vi "CH_LM VI Tree.vi"   [LabVIEW 2012, in "CH_LM.lvlib"]
doc: "This is the instrument driver for Coherent's <B>LabMax</B>. The VI Tree displays all the user-callable VIs of the instrument driver in an organized table."
uses:
  CH_LM.lvlib
  CH_LM Display Mode.ctl
  CH_LM Communication Mode.ctl
panel:
  # "(c) 2007 Coherent Inc.  ALL RIGHTS RESERVED."
  # "SEE DIAGRAM\nFOR VI TREE."
types:
  T1 = typedef "CH_LM.lvlib/CH_LM Communication Mode.ctl" = enum16{"None", "USB", "GPIB", "RS232"}
  T2 = typedef "CH_LM.lvlib/CH_LM Display Mode.ctl" = enum16{"Non-Statistics", "Statistics", "Position Stability", "Tune", "Trend"}
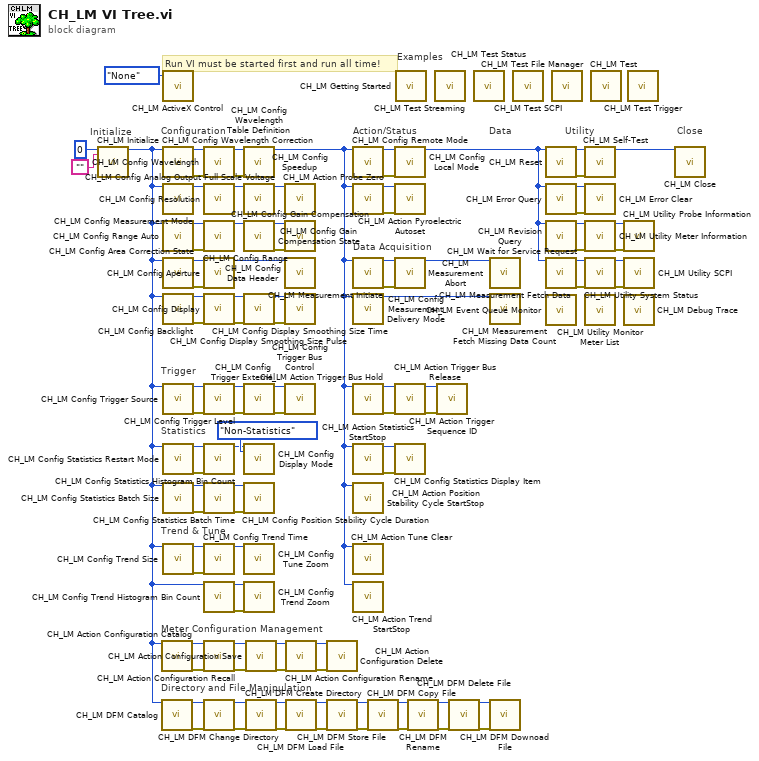
[diagram p0: block diagram]
diagram:
  # "Data Acquisition"
  # "Trigger"
  # "Statistics"
  # "Trend & Tune"
  # "Directory and File Manipulation"
  # "Meter Configuration Management"
  # "Run VI must be started first and run all time!"
  # "Examples"
  # "Configuration"
  # "Utility"
  # "Data"
  # "Action/Status"
  # "Close"
  # "Initialize"
  n1 = call "CH_LM Initialize.vi"("Address"=0, "Serial Number"="") -> ("Meter Index"=w5:i32)  [unwired: 3 in, 14 out]
  n2 = call "CH_LM Action Configuration Catalog.vi"("Meter Index"=w5) -> ("Meter Index"=w61:i32, "error out"=w60:errorcluster)  [unwired: 1 in, 16 out]
  n3 = call "CH_LM DFM Catalog.vi"("Meter Index"=w5) -> ("Meter Index"=w27:i32, "error out"=w24:errorcluster)  [unwired: 1 in, 16 out]
  n4 = call "CH_LM ActiveX Control.vi"("Communication Mode"=CH_LM_Communication_Mode."None") -> ()  [unwired: 3 in, 2 out]
  n5 = call "CH_LM Config Wavelength Correction.vi"("Meter Index"=w5) -> ("Meter Index"=w76:i32, "error out"=w9:errorcluster)  [unwired: 3 in, 14 out]
  n6 = call "CH_LM Config Measurement Mode.vi"("Meter Index"=w5) -> ("Meter Index"=w63:i32)  [unwired: 4 in, 14 out]
  n7 = call "CH_LM Config Range Auto.vi"("Meter Index"=w5) -> ("Meter Index"=w37:i32, "error out"=w11:errorcluster)  [unwired: 3 in, 14 out]
  n8 = call "CH_LM Config Area Correction State.vi"("Meter Index"=w5) -> ("Meter Index"=w73:i32, "error out"=w72:errorcluster)  [unwired: 3 in, 14 out]
  n9 = call "CH_LM Config Backlight.vi"("Meter Index"=w5) -> ("Meter Index"=w79:i32, "error out"=w78:errorcluster)  [unwired: 7 in, 10 out]
  n10 = call "CH_LM Config Trigger Source.vi"("Meter Index"=w5) -> ("Meter Index"=w45:i32, "error out"=w44:errorcluster)  [unwired: 3 in, 14 out]
  n11 = call "CH_LM Config Statistics Restart Mode.vi"("Meter Index"=w5) -> ("Meter Index"=w67:i32, "error out"=w66:errorcluster)  [unwired: 3 in, 14 out]
  n12 = call "CH_LM Config Statistics Batch Size.vi"("Meter Index"=w5) -> ("Meter Index"=w64:i32, "error out"=w65:errorcluster)  [unwired: 4 in, 13 out]
  n13 = call "CH_LM Config Trend Size.vi"("Meter Index"=w5) -> ("Meter Index"=w33:i32, "error out"=w7:errorcluster)  [unwired: 4 in, 13 out]
  n14 = call "CH_LM Config Wavelength.vi"("Meter Index"=w76, "error in (no error)"=w9) -> ("Meter Index"=w70:i32, "error out"=w10:errorcluster)  [unwired: 3 in, 13 out]
  n15 = call "CH_LM Config Resolution.vi"("Meter Index"=w63) -> ("Meter Index"=w31:i32)  [unwired: 4 in, 14 out]
  n16 = call "CH_LM Config Range.vi"("Meter Index"=w37, "error in (no error)"=w11) -> ("Meter Index"=w32:i32)  [unwired: 3 in, 14 out]
  n17 = call "CH_LM Config Aperture.vi"("Meter Index"=w73, "error in (no error)"=w72) -> ("Meter Index"=w2:i32)  [unwired: 2 in, 15 out]
  n18 = call "CH_LM Config Display.vi"("Meter Index"=w79, "error in (no error)"=w78) -> ("Meter Index"=w4:i32, "error out"=w3:errorcluster)  [unwired: 4 in, 12 out]
  n19 = call "CH_LM Config Trigger Level.vi"("Meter Index"=w45, "error in (no error)"=w44) -> ("Meter Index"=w49:i32, "error out"=w48:errorcluster)  [unwired: 2 in, 14 out]
  n20 = call "CH_LM Config Statistics Histogram Bin Count.vi"("Meter Index"=w67, "error in (no error)"=w66) -> ("Meter Index"=w15:i32)  [unwired: 2 in, 15 out]
  n21 = call "CH_LM Config Statistics Batch Time.vi"("Meter Index"=w64, "error in (no error)"=w65) -> ("Meter Index"=w51:i32, "error out"=w50:errorcluster)  [unwired: 3 in, 13 out]
  n22 = call "CH_LM Config Trend Time.vi"("Meter Index"=w33, "error in (no error)"=w7) -> ("Meter Index"=w34:i32)  [unwired: 3 in, 14 out]
  n23 = call "CH_LM Config Trend Histogram Bin Count.vi"("Meter Index"=w5) -> ("Meter Index"=w36:i32, "error out"=w35:errorcluster)  [unwired: 3 in, 14 out]
  n24 = call "CH_LM Action Configuration Recall.vi"("Meter Index"=w61, "error in (no error)"=w60) -> ("Meter Index"=w56:i32, "error out"=w59:errorcluster)  [unwired: 1 in, 15 out]
  n25 = call "CH_LM DFM Change Directory.vi"("Meter Index"=w27, "error in (no error)"=w24) -> ("Meter Index"=w26:i32, "error out"=w25:errorcluster)  [unwired: 2 in, 14 out]
  n26 = call "CH_LM Config Wavelength Table Definition.vi"("Meter Index"=w70, "error in (no error)"=w10) -> ("Meter Index"=w1:i32)  [unwired: 3 in, 14 out]
  n27 = call "CH_LM Config Analog Output Full Scale Voltage.vi"("Meter Index"=w31) -> ("Meter Index"=w77:i32)  [unwired: 3 in, 15 out]
  n28 = call "CH_LM Config Gain Compensation State.vi"("Meter Index"=w32) -> ("Meter Index"=w75:i32, "error out"=w74:errorcluster)  [unwired: 3 in, 14 out]
  n29 = call "CH_LM Config Display Smoothing Size Pulse.vi"("Meter Index"=w4, "error in (no error)"=w3) -> ("Meter Index"=w69:i32, "error out"=w68:errorcluster)  [unwired: 2 in, 14 out]
  n30 = call "CH_LM Config Trigger External.vi"("Meter Index"=w49, "error in (no error)"=w48) -> ("Meter Index"=w47:i32, "error out"=w46:errorcluster)  [unwired: 3 in, 13 out]
  n31 = call "CH_LM Config Display Mode.vi"("Meter Index"=w15, "Display Mode"=CH_LM_Display_Mode."Non-Statistics") -> ()  [unwired: 4 in, 14 out]
  n32 = call "CH_LM Config Position Stability Cycle Duration.vi"("Meter Index"=w51, "error in (no error)"=w50) -> ()  [unwired: 2 in, 16 out]
  n33 = call "CH_LM Config Tune Zoom.vi"("Meter Index"=w34) -> ()  [unwired: 5 in, 14 out]
  n34 = call "CH_LM Config Trend Zoom.vi"("Meter Index"=w36, "error in (no error)"=w35) -> ()  [unwired: 2 in, 16 out]
  n35 = call "CH_LM Action Configuration Save.vi"("Meter Index"=w56, "error in (no error)"=w59) -> ("Meter Index"=w55:i32, "error out"=w58:errorcluster)  [unwired: 1 in, 15 out]
  n36 = call "CH_LM DFM Create Directory.vi"("Meter Index"=w26, "error in (no error)"=w25) -> ("Meter Index"=w23:i32, "error out"=w22:errorcluster)  [unwired: 1 in, 15 out]
  n37 = call "CH_LM Config Speedup.vi"("Meter Index"=w77) -> ()  [unwired: 4 in, 15 out]
  n38 = call "CH_LM Config Gain Compensation.vi"("Meter Index"=w75, "error in (no error)"=w74) -> ()  [unwired: 2 in, 16 out]
  n39 = call "CH_LM Config Data Header.vi"("Meter Index"=w2) -> ()  [unwired: 4 in, 15 out]
  n40 = call "CH_LM Config Display Smoothing Size Time.vi"("Meter Index"=w69, "error in (no error)"=w68) -> ()  [unwired: 2 in, 16 out]
  n41 = call "CH_LM Config Trigger Bus Control.vi"("Meter Index"=w47, "error in (no error)"=w46) -> ()  [unwired: 2 in, 16 out]
  n42 = call "CH_LM Action Configuration Rename.vi"("Meter Index"=w55, "error in (no error)"=w58) -> ("Meter Index"=w54:i32, "error out"=w57:errorcluster)  [unwired: 2 in, 14 out]
  n43 = call "CH_LM DFM Load File.vi"("Meter Index"=w23, "error in (no error)"=w22) -> ("Meter Index"=w21:i32, "error out"=w20:errorcluster)  [unwired: 1 in, 15 out]
  n44 = call "CH_LM Action Configuration Delete.vi"("Meter Index"=w54, "error in (no error)"=w57) -> ()  [unwired: 1 in, 17 out]
  n45 = call "CH_LM DFM Store File.vi"("Meter Index"=w21, "error in (no error)"=w20) -> ("Meter Index"=w18:i32, "error out"=w19:errorcluster)  [unwired: 1 in, 15 out]
  n46 = call "CH_LM Config Remote Mode.vi"("Meter Index"=w1) -> ("Meter Index"=w94:i32, "error out"=w88:errorcluster)  [unwired: 1 in, 16 out]
  n47 = call "CH_LM Action Probe Zero.vi"("Meter Index"=w1) -> ("Meter Index"=w39:i32, "error out"=w38:errorcluster)  [unwired: 2 in, 15 out]
  n48 = call "CH_LM Measurement Initiate.vi"("Meter Index"=w1) -> ("Meter Index"=w96:i32, "error out"=w87:errorcluster)  [unwired: 1 in, 16 out]
  n49 = call "CH_LM Config Measurement Delivery Mode.vi"("Meter Index"=w1) -> ("Meter Index"=w6:i32)  [unwired: 3 in, 15 out]
  n50 = call "CH_LM Action Trigger Bus Hold.vi"("Meter Index"=w1) -> ("Meter Index"=w43:i32, "error out"=w42:errorcluster)  [unwired: 1 in, 16 out]
  n51 = call "CH_LM Action Statistics StartStop.vi"("Meter Index"=w1) -> ("Meter Index"=w53:i32, "error out"=w52:errorcluster)  [unwired: 2 in, 15 out]
  n52 = call "CH_LM Action Position Stability Cycle StartStop.vi"("Meter Index"=w1) -> ()  [unwired: 2 in, 17 out]
  n53 = call "CH_LM Action Tune Clear.vi"("Meter Index"=w1) -> ()  [unwired: 1 in, 18 out]
  n54 = call "CH_LM Action Trend StartStop.vi"("Meter Index"=w1) -> ()  [unwired: 2 in, 17 out]
  n55 = call "CH_LM DFM Copy File.vi"("Meter Index"=w18, "error in (no error)"=w19) -> ("Meter Index"=w28:i32, "error out"=w29:errorcluster)  [unwired: 2 in, 14 out]
  n56 = call "CH_LM Config Local Mode.vi"("Meter Index"=w94, "error in (no error)"=w88) -> ("Meter Index"=w71:i32)  [unwired: 17 out]
  n57 = call "CH_LM Action Pyroelectric Autoset.vi"("Meter Index"=w39, "error in (no error)"=w38) -> ()  [unwired: 18 out]
  n58 = call "CH_LM Measurement Abort.vi"("Meter Index"=w96, "error in (no error)"=w87) -> ("Meter Index"=w8:i32)  [unwired: 17 out]
  n59 = call "CH_LM Action Trigger Bus Release.vi"("Meter Index"=w43, "error in (no error)"=w42) -> ("Meter Index"=w41:i32, "error out"=w40:errorcluster)  [unwired: 16 out]
  n60 = call "CH_LM Config Statistics Display Item.vi"("Meter Index"=w53, "error in (no error)"=w52) -> ()  [unwired: 2 in, 16 out]
  n61 = call "CH_LM Getting Started.vi"() -> ()  [unwired: 2 in, 14 out]
  n62 = call "CH_LM DFM Rename.vi"("Meter Index"=w28, "error in (no error)"=w29) -> ("Meter Index"=w14:i32, "error out"=w30:errorcluster)  [unwired: 2 in, 14 out]
  n63 = call "CH_LM Test Streaming.vi"() -> ()  [unwired: 1 out]
  n64 = call "CH_LM Action Trigger Sequence ID.vi"("Meter Index"=w41, "error in (no error)"=w40) -> ()  [unwired: 1 in, 17 out]
  n65 = call "CH_LM DFM Delete File.vi"("Meter Index"=w14, "error in (no error)"=w30) -> ("Meter Index"=w13:i32, "error out"=w17:errorcluster)  [unwired: 2 in, 14 out]
  n66 = call "CH_LM Test Status.vi"() -> ()  [unwired: 1 out]
  n67 = call "CH_LM Measurement Fetch Data.vi"("Meter Index"=w8) -> ()  [unwired: 2 in, 17 out]
  n68 = call "CH_LM Measurement Fetch Missing Data Count.vi"("Meter Index"=w6) -> ()  [unwired: 1 in, 18 out]
  n69 = call "CH_LM DFM Downoad File.vi"("Meter Index"=w13, "error in (no error)"=w17) -> ()  [unwired: 2 in, 16 out]
  n70 = call "CH_LM Test SCPI.vi"() -> ()  [unwired: 1 out]
  n71 = call "CH_LM Reset.vi"("Meter Index"=w71) -> ("Meter Index"=w97:i32, "error out"=w89:errorcluster)  [unwired: 2 in, 15 out]
  n72 = call "CH_LM Error Query.vi"("Meter Index"=w71) -> ("Meter Index"=w83:i32, "error out"=w82:errorcluster)  [unwired: 1 in, 16 out]
  n73 = call "CH_LM Revision Query.vi"("Meter Index"=w71) -> ("Meter Index"=w81:i32, "error out"=w80:errorcluster)  [unwired: 1 in, 16 out]
  n74 = call "CH_LM Wait for Service Request.vi"("Meter Index"=w71) -> ("Meter Index"=w93:i32, "error out"=w92:errorcluster)  [unwired: 1 in, 16 out]
  n75 = call "CH_LM Event Queue Monitor.vi"() -> ()  [unwired: 1 out]
  n76 = call "CH_LM Test File Manager.vi"() -> ()  [unwired: 1 out]
  n77 = call "CH_LM Self-Test.vi"("Meter Index"=w97, "error in (no error)"=w89) -> ("Meter Index"=w84:i32)  [unwired: 17 out]
  n78 = call "CH_LM Error Clear.vi"("Meter Index"=w83, "error in (no error)"=w82) -> ()  [unwired: 18 out]
  n79 = call "CH_LM Utility Meter Information.vi"("Meter Index"=w81, "error in (no error)"=w80) -> ("Meter Index"=w86:i32, "error out"=w85:errorcluster)  [unwired: 3 in, 13 out]
  n80 = call "CH_LM Utility System Status.vi"("Meter Index"=w93, "error in (no error)"=w92) -> ("Meter Index"=w91:i32, "error out"=w90:errorcluster)  [unwired: 16 out]
  n81 = call "CH_LM Utility Monitor Meter List.vi"() -> ()  [unwired: 1 out]
  n82 = call "CH_LM Test.vi"() -> ()  [unwired: 1 out]
  n83 = call "CH_LM Utility Probe Information.vi"("Meter Index"=w86, "error in (no error)"=w85) -> ()  [unwired: 18 out]
  n84 = call "CH_LM Utility SCPI.vi"("Meter Index"=w91, "error in (no error)"=w90) -> ()  [unwired: 2 in, 16 out]
  n85 = call "CH_LM Debug Trace.vi"() -> ()  [unwired: 1 out]
  n86 = call "CH_LM Test Trigger.vi"() -> ()  [unwired: 1 out]
  n87 = call "CH_LM Close.vi"("Meter Index"=w84) -> ()  [unwired: 1 in, 18 out]
